vi "845x_I2C Write.vi"(0 "Device":T1, 1 "Address":u16=80 format="%.0x", 2 "Clock Rate (kHz)":u16=100, 3 "EEPROM Data Address":u16 format="%.0x", 4 "Data to Write":u8[](array[numeric]), 5 "error in (no error)":errorcluster, 6 "I/O Voltage Level":i32(ring)=33 items=["3.3V"=33, "2.5V"=25, "1.8V"=18, "1.5V"=15, "1.2V"=12], 7 "Data Address Width":enum16{"1 Byte", "2 Byte"}(ring)=enum."2 Byte", 8 "Use Internal I2C Pullup Resistor":bool, 9 "Data Address Endianness":bool=TRUE, 11 "Target Page Size (bytes)":u32=128, 13 "Write Delay Between Pages (ms)":u32=4) -> (19 "error out":errorcluster)   [LabVIEW 2021, in "Communication.lvlib"]
doc: "<B>NOTE: This example is taken from ni845x driver examples located at C:\\Program Files (x86)\\National Instruments\\LabVIEW <version>\\examples\\ni845x\\845xEx.llb. More such examples can be found in the same location.</B>\n\nThis EEPROM example shows a more generalized way to use the I2C basic API to write data. It allows the user to change the following parameters: page size, write delay, the endianness of the address bytes, and the number of bytes in an address.\n\nThe parameters will have the following effects:\n\nTarget Page Size (bytes): This places an additional constraint on the amount of bytes written. The smaller value will be used, and that number of bytes written.\nWrite Delay Between Pages (ms): This will force a mandatory delay after writing bytes to a device.\nData Address Width: This will allow the user to specify the EEPROM Data Address as either 1 or 2 bytes.\nData Address Endianness: This control will change the ordering of the bytes in the EEPROM Data Address, note that this only has an effect if there are 2 bytes in the address.\n\nSince the I2C SDA and SCL lines are open-drain, they must be pulled up to the required reference voltage of your slave by connecting an appropriate resistor (2k-5k) between SCL and your reference voltage and SDA and your reference voltage. For NI-845x Hardware that contain internal pull-ups, you can use these. Otherwise, you need to use external pullups.\n\nFor connection information see the NI-845x Hardware and Software manual and the manual for your specific EEPROM."
uses:
  Communication.lvlib
  <vilib>/ni845x/ni845x.llb/ni845xControl.ctl
  <vilib>/ni845x/ni845x.llb/NI-845x I2C Close Configuration Reference.vi
  <resource>/objmgr/NI845x.rc
panel:
  # "See VI Info <Ctrl+I> for more information on how to use this example"
  # "Device Configuration"
  # "I2C Slave Configuration"
  # "I2C Data"
  # "Big Endian"
  # "Little Endian"
  # "NOTE: This example is taken from ni845x driver examples located at C:\\Program Files (x86)\\National Instruments\\LabVIEW <version>\\examples\\ni845x\\845xEx.llb. More such examples can be found in the same location."
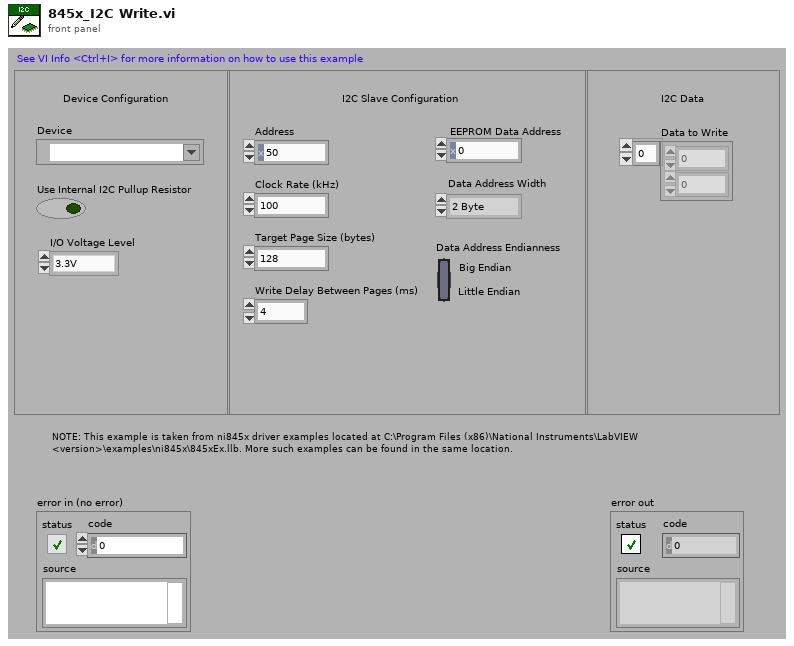
[diagram p1: front panel]
types:
  T1 = typedef "ni845xControl.ctl" = refnum<k21>
  T2 = typedef "ni845xI2cConfiguration.ctl" = refnum<k20>
  T3 = cluster{"EEPROM Address":u16, "Length":u32, "Data Index":u32}[]
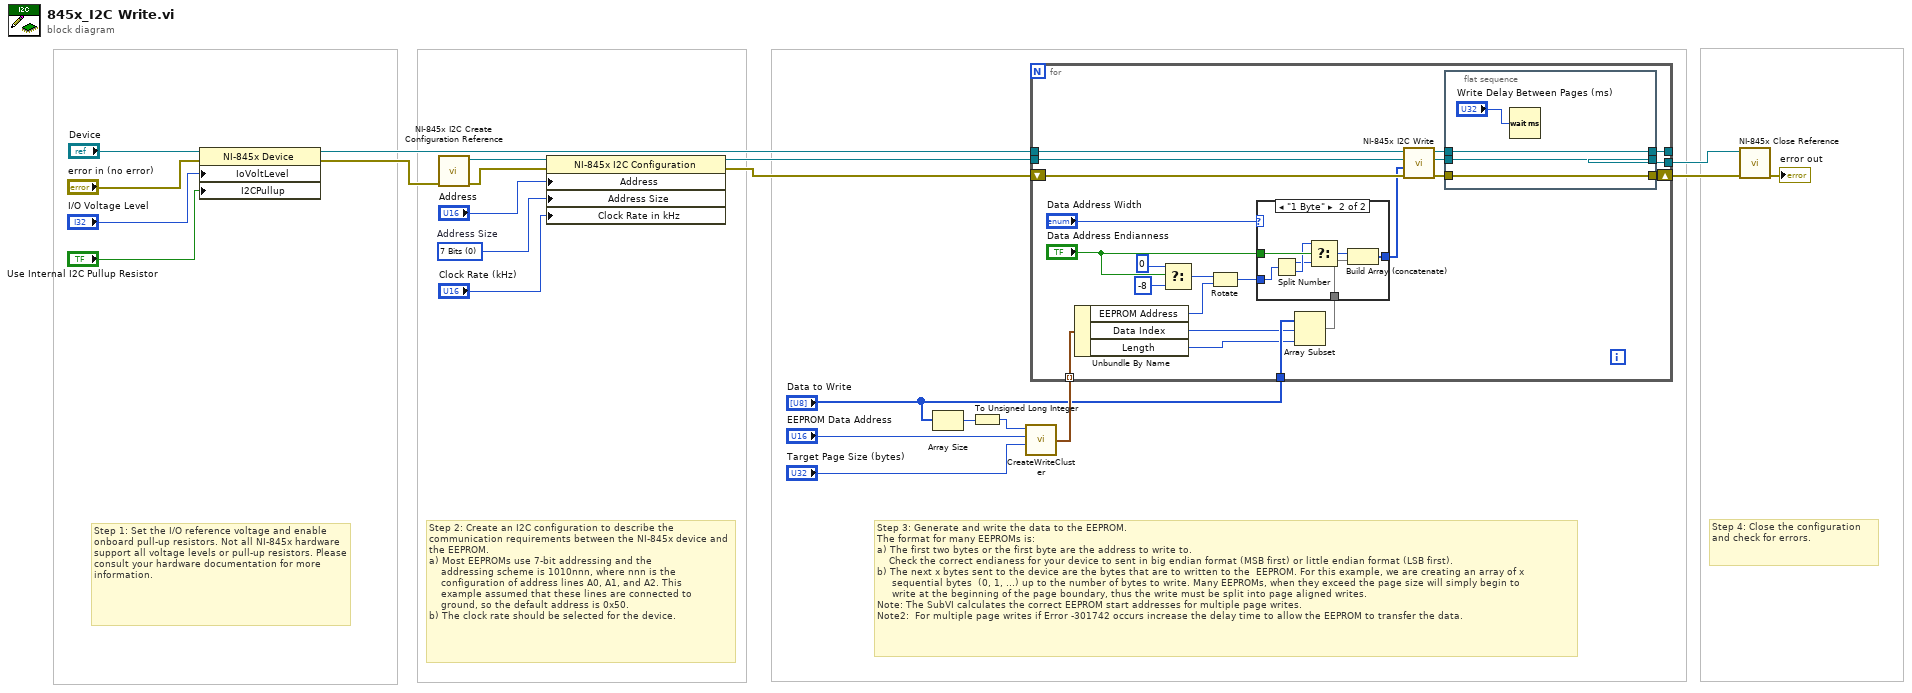
[diagram p0: block diagram]
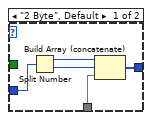
[diagram p2: hidden frame]
diagram:
  w21 = 0 items=["7 Bits", "10 Bits"]  # Address Size
  # "Step 1: Set the I/O reference voltage and enable onboard pull-up resistors. Not all NI-845x hardware support all voltage levels or pull-up resistors. Please consult your hardware documentation for more information."
  # "Step 4: Close the configuration \nand check for errors."
  # "Step 2: Create an I2C configuration to describe the \ncommunication requirements between the NI-845x device and the EEPROM.\na) Most EEPROMs use 7-bit addressing and the\n    addressing scheme is 1010nnn, where nnn is the\n    configuration of address lines A0, A1, and A2. This    \n    example assumed that these lines are connected to\n    ground, so the default address is 0x50. \nb) The clock rate should be selected for the device."
  # "Step 3: Generate and write the data to the EEPROM. \nThe format for many EEPROMs is:\na) The first two bytes or the first byte are the address to write to. \n    Check the correct endianess for your device to sent in big endian format (MSB first) or little endian format (LSB first).\nb) The next x bytes sent to the device are the bytes that are to written to the  EEPROM. For this example, we are creating an array of x\n     sequential bytes  (0, 1, ...) up to the number of bytes to write. Many EEPROMs, when they exceed the page size will simply begin to\n     write at the beginning of the page boundary, thus the write must be split into page aligned writes.\nNote: The SubVI calculates the correct EEPROM start addresses for multiple page writes.\nNote2:  For multiple page writes if Error -301742 occurs increase the delay time to allow the EEPROM to transfer the data."
  n1 = property on="Property Node" class="NI-845x Device"(reference="Device", error in="error in (no error)", "IoVoltLevel"="I/O Voltage Level", "I2CPullup"="Use Internal I2C Pullup Resistor") -> (reference out=w9:T1, error out=w8:errorcluster)
  n2 = call <vilib>:"NI-845x I2C Create Configuration Reference.vi"("error in (no error)"=w8) -> ("error out"=w18:errorcluster, "i2c configuration"=w19:T2)  [unwired: 9 out]
  n3 = property on="Property Node" class="NI-845x I2C Configuration"(reference=w19, error in=w18, "Address"="Address", "Address Size"=w21, "Clock Rate in kHz"="Clock Rate (kHz)") -> (reference out=w16:T2, error out=w15:errorcluster)
  n4 = Array Size(array="Data to Write") -> (size(s)=w2:i32)
  n5 = To Unsigned Long Integer(number=w2) -> (unsigned 32bit integer=w1:u32)
  n6 = call "CreateWriteCluster.vi"("Page Size in Bytes"="Target Page Size (bytes)", "EEPROM Starting Address"="EEPROM Data Address", "Number of Bytes to Write"=w1) -> ("Array of Write Cluster Information"=w11:T3)  [unwired: 1 out]
  n7 = for {
    shift-right: [w44] -> w17
    shift-left: w15 -> [w41]
    tunnel: "Data to Write" -> [w27]
    tunnel: w9 -> [w39]
    tunnel: [w43] -> _
    tunnel: w16 -> [w42]
    tunnel: [w30] -> w14
    tunnel: w11 -> [w23] mode=indexing
    n8 = Unbundle By Name(w23) -> ("EEPROM Address"=w24:u16, "Data Index"=w25:u32, "Length"=w26:u32)
    n9 = Select(t=i16 0, s="Data Address Endianness", f=i16 -8) -> (s? t:f=w35:i16)
    n10 = Rotate(1:w24, 2:w35) -> (0:w34:u16)
    n11 = Array Subset(array=w27, index=w25, length=w26) -> (w29:u8[])
    n12 = case shown="\"1 Byte\"" "Data Address Width" {
      tunnel: w34 -> [w49 w54]
      tunnel: [w48 w56] -> w32
      tunnel: w29 -> [w47 w55]
      tunnel: "Data Address Endianness" -> [_ w53]
      frame "2 Byte", Default {
        n13 = Split Number(x=w49) -> (hi(x)=w45:u8, lo(x)=w46:u8)
        n14 = Build Array (concatenate)(w45, w46, w47) -> (w48:u8[])
      }
      frame "1 Byte" {
        n15 = Split Number(x=w54) -> (hi(x)=w50:u8, lo(x)=w51:u8)
        n16 = Select(t=w51, s=w53, f=w50) -> (s? t:f=w52:u8)
        n17 = Build Array (concatenate)(w52, w55) -> (w56:u8[])
      }
    }
    n18 = call <vilib>:"NI-845x I2C Write.vi"("error in (no error)"=w41, "write data"=w32, "i2c configuration in"=w42, "device reference in"=w39) -> ("error out"=w40:errorcluster, "i2c configuration out"=w31:T2, "device reference out"=w38:T1)  [unwired: 5 out]
    n19 = flat-sequence {
      tunnel: [w60] -> w44
      tunnel: [w59] -> w43
      tunnel: w38 -> [w59]
      tunnel: w40 -> [w60]
      tunnel: w31 -> [w58]
      tunnel: [w58] -> w30
      frame #0 {
        n20 = Wait (ms)(milliseconds to wait="Write Delay Between Pages (ms)") -> ()  [unwired: 1 out]
      }
    }
  }
  n21 = call-poly <vilib>:"NI-845x Close Reference.vi"("error in (no error)"=w17, "i2c configuration"=w14) -> ("error out"=→"error out":errorcluster)  [unwired: 9 out]
